vi "CRYASIOGetDeviceCount.vi"(9 "InOut":bool=TRUE, 10 "Driver Name":string, 11 "error in (no error)":errorcluster) -> (2 "Device Count":u32, 3 "error out":errorcluster)   [LabVIEW 2013]
uses:
  CRY_ASIO.dll
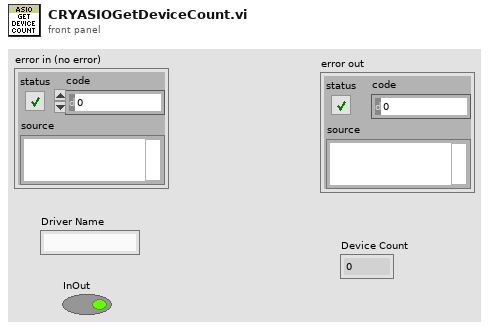
[diagram p1: front panel]
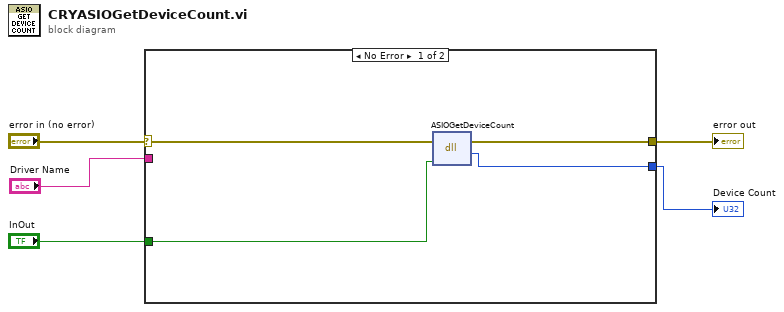
[diagram p0: block diagram]
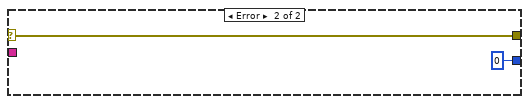
[diagram p2: hidden frame]
diagram:
  n1 = case shown="No Error" "error in (no error)" {
    selector: "error in (no error)" -> [w6 w11]
    tunnel: "Driver Name" -> [_ _]
    tunnel: [w9 w11] -> w3
    tunnel: [w8 u32 0 ("return type")] -> w2
    tunnel: "InOut" -> [w7 _]
    frame No Error {
      n2 = dll-call lib="D:/LabView_Project/CRY6181/CRY_ASIO.dll" fn="ASIOGetDeviceCount"(error in=w6, "arg1"=w7) -> (error out=w9:errorcluster, "return type"=w8:u32)  [unwired: 3 in, 1 out]
    }
    frame Error {
    }
  }
  "error out" <- w3
  "Device Count" <- w2
